vi "outputs to tagbus.vi"(9 "output in":dbl[](array[numeric]), 10 "Processing Outputs":T2, 11 "tag bus in":T1) -> (3 "tag bus out":T1)   [LabVIEW 2013, in "PID Module runtime.lvclass"]
uses:
  PID Module runtime.lvclass
  <vilib>/NI/Tag Bus/table/data table.ctl
  processing outputs.ctl
  <vilib>/NI/Tag Bus/table/data polymorphs/write one/write Double.vi
  <vilib>/NI/Tag Bus/table/data table.lvlib
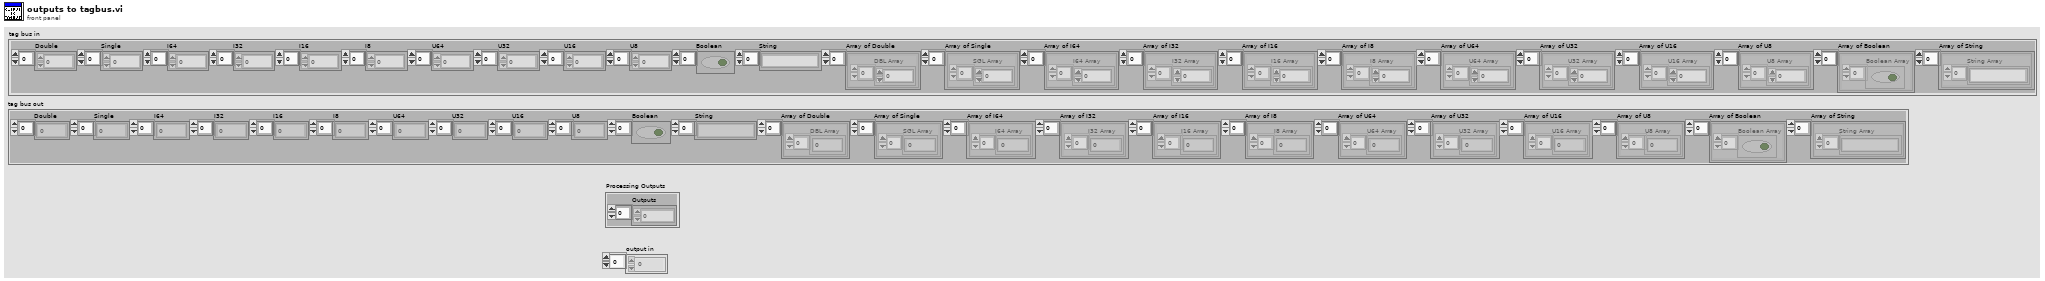
[diagram p1: front panel]
types:
  T1 = typedef "tag bus.lvlib/data table.lvlib/data table.ctl" = cluster{"Double":dbl[], "Single":sgl[], "I64":i64[], "I32":i32[], "I16":i16[], "I8":i8[], "U64":u64[], "U32":u32[], "U16":u16[], "U8":u8[], "Boolean":bool[], "String":string[], "Array of Double":cluster{"DBL Array":dbl[]}[], "Array of Single":cluster{"SGL Array":sgl[]}[], "Array of I64":cluster{"I64 Array":i64[]}[], "Array of I32":cluster{"I32 Array":i32[]}[], "Array of I16":cluster{"I16 Array":i16[]}[], "Array of I8":cluster{"I8 Array":i8[]}[], "Array of U64":cluster{"U64 Array":u64[]}[], "Array of U32":cluster{"U32 Array":u32[]}[], "Array of U16":cluster{"U16 Array":u16[]}[], "Array of U8":cluster{"U8 Array":u8[]}[], "Array of Boolean":cluster{"Boolean Array":bool[]}[], "Array of String":cluster{"String Array":string[]}[]}
  T2 = typedef "PID Module runtime.lvclass/processing outputs.ctl" = cluster{"Outputs":i32[]}
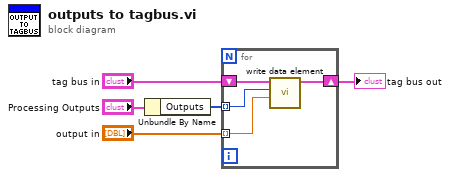
[diagram p0: block diagram]
diagram:
  n1 = Unbundle By Name("Processing Outputs") -> ("Outputs"=w1:i32[])
  n2 = for {
    shift-right: [w8] -> w4
    shift-left: "tag bus in" -> [w9]
    tunnel: "output in" -> [w7] mode=indexing
    tunnel: w1 -> [w6] mode=indexing
    n3 = call-poly <vilib>:"write data element.vi"("value"=w7, "index"=w6, "data table in"=w9) -> ("data table out"=w8:T1)  [unwired: 8 in]
  }
  "tag bus out" <- w4
